vi "Output Enable Write Array.vi"(8 "error in":errorcluster, 9 "Number of Channels":u32=1, 10 "Output Enable STS":i32[](array[numeric]), 11 "Output Enable in":refnum<class "Output Enable.lvclass">) -> (0 "error out":errorcluster, 3 "Output Enable out":refnum<class "Output Enable.lvclass">)   [LabVIEW 2023, in "Output Enable.lvclass"]
uses:
  Output Enable.lvclass
  Output Enable.lvclass/Output Enable.ctl
  <vilib>/ADAS Replay HIL/Channels/Tag Wrapper/Polymorphic/Write Channel (I32).vi
  <vilib>/ADAS Replay HIL/Channels/Tag Wrapper/Polymorphic/Write Channel (I32).vi/cccb8e89-591f-4bb4-9d4e-ae06ba1f5498.vi
  <vilib>/ADAS Replay HIL/Channels/Tag Wrapper/Polymorphic/Write Channel (I32).vi/cccb8e89-591f-4bb4-9d4e-ae06ba1f5498.vi/4bc1c15b-36ab-481f-b8dd-c64075ce723a.vi
  <vilib>/ADAS Replay HIL/Channels/Tag Wrapper/Polymorphic/Write Channel (I32).vi/cccb8e89-591f-4bb4-9d4e-ae06ba1f5498.vi/d83cb72b-7713-41fc-a3d1-682de79cf574.vi
  <vilib>/ADAS Replay HIL/Channels/Tag Wrapper/Tag Wrapper.lvlib
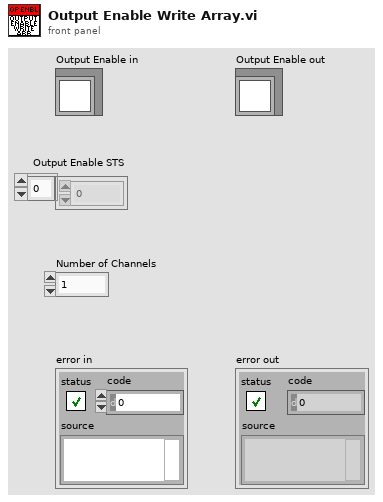
[diagram p1: front panel]
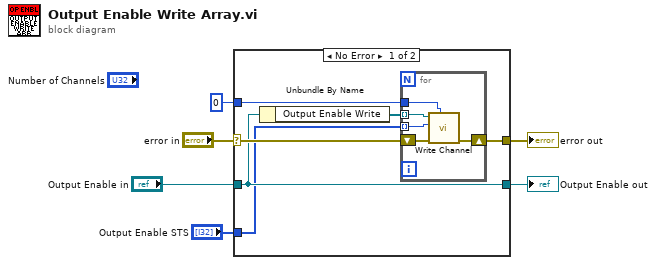
[diagram p0: block diagram]
diagram:
  n1 = case shown="No Error" "error in" {
    selector: "error in" -> [w12 w19]
    tunnel: [w11 w19] -> w5
    tunnel: [w9 w18] -> w3
    tunnel: "Output Enable in" -> [w9 w18]
    tunnel: "Output Enable STS" -> [w8 _]
    tunnel: 0 ("Timeout (ms)") -> [w7 _]
    frame No Error {
      n2 = Unbundle By Name(w9) -> ("Output Enable Write"=w10:refnum<k21>[])
      n3 = for {
        shift-right: [w16] -> w11
        shift-left: w12 -> [w17]
        tunnel: w10 -> [w15] mode=indexing
        tunnel: w8 -> [w14] mode=indexing
        tunnel: w7 -> [w13]
        n4 = call-poly <vilib>:"Write Channel.vi"("Timeout (ms)"=w13, "error in"=w17, "Value to Write"=w14, "ADAS HIL Channel in"=w15) -> ("error out"=w16:errorcluster)  [unwired: 5 in, 2 out]
      }
    }
    frame Error {
    }
  }
  "error out" <- w5
  "Output Enable out" <- w3
